vi "Query Voltage Unit.vi"(8 "error in (no error)":errorcluster, 10 "Channel (0: Channel 1)":T2 items=["Channel 1", "Channel 2"], 11 "VISA resource name":refnum<visa-resource-name>) -> (0 "error out":errorcluster, 1 "Volt Unit":T1, 3 "VISA resource name out":refnum<visa-resource-name>)   [LabVIEW 2009, in "Tektronix AFG 3000 Series.lvlib"]
doc: "Queries the units used when setting the voltage amplitude of a Tektronix AFG 3000 series function generator. (This setting does not affect the offest, high, or low voltage commands.)"
uses:
  Tektronix AFG 3000 Series.lvlib
  controls.llb/Channel.ctl
  controls.llb/Volt Unit.ctl
  <vilib>/Utility/error.llb/DialogType.ctl
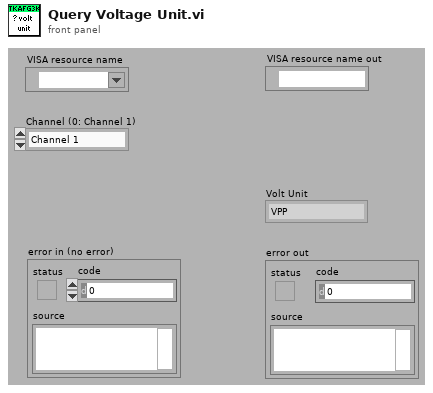
[diagram p1: front panel]
types:
  T1 = typedef "Volt Unit.ctl" = enum16{"VPP", "VRMS", "DBM"}
  T2 = typedef "Channel.ctl" = u16
  T3 = typedef "DialogType.ctl" = u16
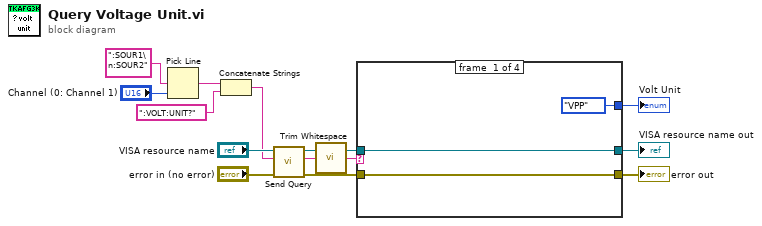
[diagram p0: block diagram]
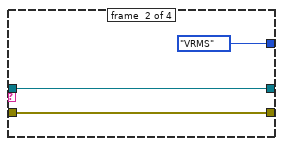
[diagram p2: hidden frame]
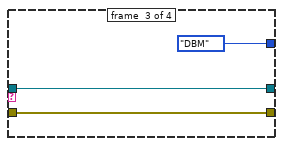
[diagram p3: hidden frame]
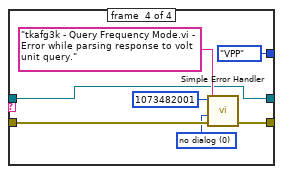
[diagram p4: hidden frame]
diagram:
  n1 = Pick Line(multi-line string=":SOUR1\n:SOUR2", line index="Channel (0: Channel 1)") -> (output string=w11:string)  [unwired: 1 out]
  n2 = Concatenate Strings(w11, ":VOLT:UNIT?" ("format string")) -> (w10:string)
  n3 = call "Send Query.vi"("error in (no error)"="error in (no error)", "write buffer"=w10, "VISA resource name"="VISA resource name") -> ("error out"=w7:errorcluster, "read buffer"=w3:string, "VISA resource name out"=w6:refnum<visa-resource-name>)  [unwired: 1 in, 5 out]
  n4 = call <vilib>:"Trim Whitespace.vi"("string"=w3) -> ("trimmed string"=w2:string)  [unwired: 1 in]
  n5 = case shown="\"DBM\"" w2 {
    tunnel: [Volt_Unit."VPP" ("Volt Unit (VPP)") Volt_Unit."VRMS" ("Volt Unit (VPP)") Volt_Unit."DBM" ("Volt Unit (VPP)") Volt_Unit."VPP" ("Volt Unit (VPP)")] -> w1
    tunnel: w7 -> [w16 w19 w22 w30]
    tunnel: w6 -> [w17 w20 w23 w25]
    tunnel: [w17 w20 w23 w25] -> w5
    tunnel: [w16 w19 w22 w29] -> w4
    frame #0 {
    }
    frame #1 {
    }
    frame #2 {
    }
    frame #3 {
      w28 = T3 0 items=["no dialog", "OK message", "continue or stop message", "OK message + warnings", "continue/stop + warnings"] ("type of dialog (OK msg:1)")
      n6 = call <vilib>:"Simple Error Handler.vi"("error code (no error:0)"=1073482001, "error source (\" \")"="tkafg3k - Query Frequency Mode.vi - Error while parsing response to volt unit query." ("error source (\" \")"), "type of dialog (OK msg:1)"=w28, "error in (no error)"=w30) -> ("error out"=w29:errorcluster)  [unwired: 5 out]
    }
  }
  "error out" <- w4
  "VISA resource name out" <- w5
  "Volt Unit" <- w1
